vi "QTrkReadTimestampFromFramePtr.vi"(9 "height":i32, 10 "width":i32, 11 "imageptr":u64) -> (3 "timestamp":u32)   [LabVIEW 2011]
uses:
  QTrkDLL.vi
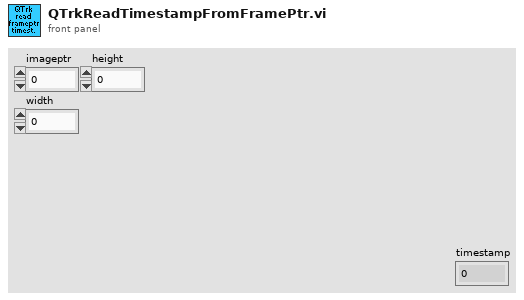
[diagram p1: front panel]
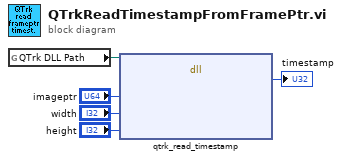
[diagram p0: block diagram]
diagram:
  n1 = global read "QTrkDLL.vi" "QTrk DLL Path"() -> (w5:path)
  n2 = dll-call lib="D:/jcnossen1/cudaqi-tracker/bin/jtrkcuda-labview.dll" fn="qtrk_read_timestamp"(path in=w5, "imageptr"="imageptr", "width"="width", "height"="height") -> ("timestamp"=→"timestamp":u32)  [unwired: 5 in, 2 out]
